vi "Update PhXP Parameters.vi"(8 "error in (no error)":errorcluster, 11 "VI in":refnum<vi>) -> (0 "error out":errorcluster, 2 "tau*":dbl[unit], 3 "f0":dbl[unit])   [LabVIEW 2019]
uses:
  Phasor Explorer Phasor Parameters.ctl
  Phasor Calculation Type.ctl
  Phasor Type.ctl
  Phasor Explorer Gate Parameters.ctl
  Gate Type.ctl
  SEPXP Gate Parameter to Adjust.ctl
  Phasor Explorer Decay Parameters.ctl
  IRF Model.ctl
  Phasor Explorer Display Parameters.ctl
  Type of Series.ctl
panel:
  in  "Edit User-defined Gate":bool
  in  "Phasor Explorer Display Parameters":T1={"# Points"=1, "Ramp Type"=enum."Linear", "Type of Series"=enum."1-Exp Decays", "Min tau"=0.0, "Max tau"=0.0, "Include 0"=FALSE, "Include Infinity"=FALSE} {"Min tau" min=0.0; "Max tau" min=0.0; "# Points" min=1 step=1}
  in  "Phasor Explorer Decay & IRF Parameters":T3 {"Lifetime" min=0.0; "Laser Period" min=0.0}
  in  "Gate Parameter to Adjust":T5 caption="Parameter to adjust"
  in  "Phasor Explorer Gate Parameters":T6={"First Gate Start"=0.0, "Use Gate Center"=FALSE, "Gate Width"=0.0, "Gate Step"=0.0, "# Gates"=1.0, "Gate Type"=enum."Square", "Edge Width"=0.0, "Top Slope"=0.0, "Reversed Sawtooth?"=FALSE, "Analytical Computation"=FALSE, "Tolerance"=1.0, "Integration"=enum."Item 0", "# Steps"=1.0, "Type of User-defined Function"=enum."Gate"} {"# Steps" min=0.0; "Tolerance" min=0.0; "Top Slope" min=0.0; "Edge Width" min=0.0; "Gate Step" min=0.0; "# Gates" min=1.0 step=1.0; "Gate Width" min=0.0}
  in  "Phasor Explorer Phasor Parameters":T8={"Harmonic frequency"=0.0, "Use f* = 1/D Frequency"=FALSE, "Calibrated Phasor"=FALSE, "Calibration Lifetime"=1e-09, "Phasor Calculation"=enum."Direct Sum", "SEPL Type"=enum."UC", "# Gates"=1.0, "Square Gate Width"=1e-09, "Show Ticks"=FALSE} {"Square Gate Width" min=0.0; "# Gates" min=0.0; "Calibration Lifetime" min=0.0; "Harmonic frequency" min=0.0}
  in  "Match Laser Period":bool
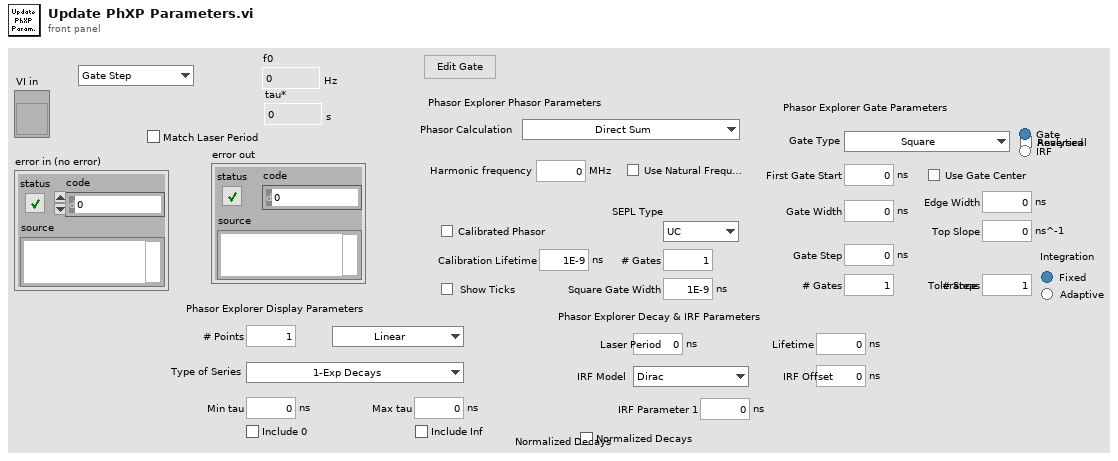
[diagram p1: front panel]
types:
  T1 = typedef "Phasor Explorer Display Parameters.ctl" = cluster{"# Points":i32, "Ramp Type":enum16{"Linear", "Logarithmic"}, "Type of Series":T2, "Min tau":dbl[unit], "Max tau":dbl[unit], "Include 0":bool, "Include Infinity":bool}
  T2 = typedef "Type of Series.ctl" = enum16{"1-Exp Decays", "Linear Combination of 1-Exp"}
  T3 = typedef "Phasor Explorer Decay Parameters.ctl" = cluster{"Lifetime":dbl[unit], "IRF Offset":dbl[unit], "Laser Period":dbl[unit], "Normalized Decays":bool, "IRF Model":T4, "IRF Parameter 1":dbl[unit]}
  T4 = typedef "IRF Model.ctl" = enum16{"Dirac", "Exponential"}
  T5 = typedef "SEPXP Gate Parameter to Adjust.ctl" = enum16{"Gate Step", "# Gates"}
  T6 = typedef "Phasor Explorer Gate Parameters.ctl" = cluster{"First Gate Start":dbl[unit], "Use Gate Center":bool, "Gate Width":dbl[unit], "Gate Step":dbl[unit], "# Gates":dbl, "Gate Type":T7, "Edge Width":dbl[unit], "Top Slope":dbl[unit], "Reversed Sawtooth?":bool, "Analytical Computation":bool, "Tolerance":dbl, "Integration":enum32{"Item 0", "Item 1"}, "# Steps":dbl, "Type of User-defined Function":enum32{"Gate", "IRF"}}
  T7 = typedef "Gate Type.ctl" = enum16{"Square", "Finite Edge Square", "Finite Edge, Tilted Top Square", "Triangle", "Sawtooth", "User-defined"}
  T8 = typedef "Phasor Explorer Phasor Parameters.ctl" = cluster{"Harmonic frequency":dbl[unit], "Use f* = 1/D Frequency":bool, "Calibrated Phasor":bool, "Calibration Lifetime":dbl[unit], "Phasor Calculation":T9, "SEPL Type":T10, "# Gates":dbl, "Square Gate Width":dbl[unit], "Show Ticks":bool}
  T9 = typedef "Phasor Calculation Type.ctl" = enum16{"Direct Sum", "Analytical Formula"}
  T10 = typedef "Phasor Type.ctl" = enum16{"UC", "L_N", "L_N[W]"}
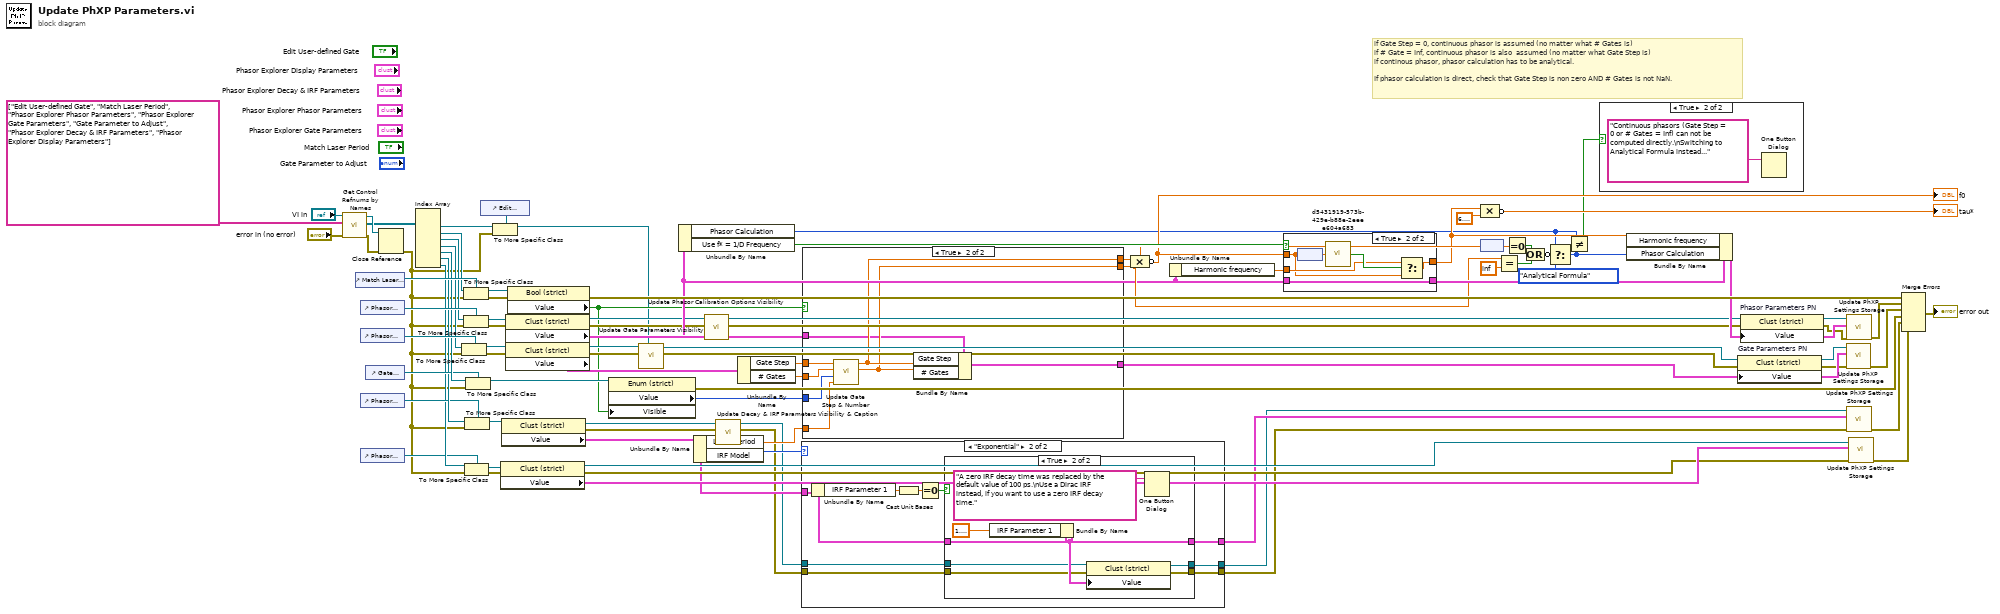
[diagram p0: block diagram]
diagram:
  # "if Gate Step = 0, continuous phasor is assumed (no matter what # Gates is)\nif # Gate = Inf, continuous phasor is also  assumed (no matter what Gate Step is)\nif continous phasor, phasor calculation has to be analytical.\n\nIf phasor calculation is direct, check that Gate Step is non zero AND # Gates is not NaN."
  n1 = call "Get Control Refnums by Names.vi"("error in"="error in (no error)", "Control Labels"=string[] ["Edit User-defined Gate", "Match Laser Period", "Phasor Explorer Phasor Parameters", "Phasor Explorer Gate Parameters", "Gate Parameter to Adjust", "Phasor Explorer Decay & IRF Parameters", "Phasor Explorer Display Parameters"], "VI  Ref"="VI in") -> ("error out"=w5:errorcluster, "Ctl Refnums"=w86:refnum<vi>[], "VI  Ref (out)"=w87:refnum<vi>)  [unwired: 5 in, 1 out]
  n2 = control-ref of="Match Laser Period"() -> (w79:refnum<vi>)
  n3 = control-ref of="Phasor Explorer Phasor Parameters"() -> (w82:refnum<vi>)
  n4 = control-ref of="Phasor Explorer Gate Parameters"() -> (w81:refnum<vi>)
  n5 = control-ref of="Phasor Explorer Decay & IRF Parameters"() -> (w54:refnum<vi>)
  n6 = control-ref of="Phasor Explorer Display Parameters"() -> (w33:refnum<vi>)
  n7 = control-ref of="Gate Parameter to Adjust"() -> (w73:refnum<vi>)
  n8 = Close Reference(reference=w87, error in (no error)=w5) -> (error out=w2:errorcluster)
  n9 = Index Array(array=w86) -> (element #1=w4:refnum<vi>, element #2=w58:refnum<vi>, element #3=w57:refnum<vi>, element #4=w56:refnum<vi>, element #5=w75:refnum<vi>, element #6=w55:refnum<vi>, element #7=w34:refnum<vi>)  [unwired: 7 in]
  n10 = To More Specific Class(target class=w81, reference=w56, error in=w2) -> (specific class reference=w62:refnum<vi>, error out=w61:errorcluster)
  n11 = To More Specific Class(target class=w79, reference=w58, error in=w2) -> (specific class reference=w78:refnum<vi>, error out=w77:errorcluster)
  n12 = To More Specific Class(target class=w82, reference=w57, error in=w2) -> (specific class reference=w64:refnum<vi>, error out=w63:errorcluster)
  n13 = To More Specific Class(target class=w33, reference=w34, error in=w2) -> (specific class reference=w32:refnum<vi>, error out=w31:errorcluster)
  n14 = To More Specific Class(target class=w54, reference=w55, error in=w2) -> (specific class reference=w53:refnum<vi>)  [unwired: 1 out]
  n15 = To More Specific Class(target class=w73, reference=w75, error in=w2) -> (specific class reference=w74:refnum<vi>)  [unwired: 1 out]
  n16 = control-ref of="Edit User-defined Gate"() -> (w3:refnum<vi>)
  n17 = To More Specific Class(target class=w3, reference=w4, error in=w2) -> (specific class reference=w1:refnum<vi>)  [unwired: 1 out]
  n18 = property class="Clust (strict)"(reference=w32, error in=w31) -> (reference out=w28:refnum<vi>, error out=w26:errorcluster, "Value"=w27:T1)
  n19 = property class="Clust (strict)"(reference=w53) -> (reference out=w22:refnum<vi>, error out=w8:errorcluster, "Value"=w24:T3)  [unwired: 1 in]
  n20 = property class="Clust (strict)"(reference=w64, error in=w63) -> (reference out=w16:refnum<vi>, error out=w14:errorcluster, "Value"=w42:T8)
  n21 = property class="Clust (strict)"(reference=w62, error in=w61) -> (reference out=w35:refnum<vi>, error out=w12:errorcluster, "Value"=w51:T6)
  n22 = property class="Bool (strict)"(reference=w78, error in=w77) -> (error out=w76:errorcluster, "Value"=w6:bool)  [unwired: 1 out]
  n23 = property class="Enum (strict)"(reference=w74, "Visible"=w6) -> (error out=w71:errorcluster, "Value"=w72:T5)  [unwired: 1 in, 1 out]
  n24 = call "Update Gate Parameters Visibility.vi"("Edit User-defined Gate"=w1, "error in (no error)"=w12, "Phasor Explorer Gate Parameters in"=w35) -> ("error out"=w11:errorcluster, "Phasor Explorer Gate Parameters out"=w10:refnum<vi>)  [unwired: 7 in]
  n25 = Unbundle By Name(w42) -> ("Phasor Calculation"=w19:T9, "Use f* = 1/D Frequency"=w85:bool)
  n26 = Unbundle By Name(w24) -> ("Laser Period"=w52:dbl[unit], "IRF Model"=w25:T4)
  n27 = call "Update Phasor Calibration Options Visibility.vi"("Error In"=w14, "Phasor Explorer Phasor Parameters Refnum in"=w16) -> ("Error Out"=w13:errorcluster, "Phasor Explorer Phasor Parameters Refnum out"=w15:refnum<vi>)  [unwired: 8 in]
  n28 = call "Update Decay & IRF Parameters Visibility & Caption.vi"("error in (no error)"=w8, "Phasor Explorer Decay & IRF Parameters in"=w22) -> ("error out"=w7:errorcluster, "Phasor Explorer Decay & IRF Parameters out"=w9:refnum<vi>)  [unwired: 8 in]
  n29 = Unbundle By Name(w51) -> ("Gate Step"=w60:dbl[unit], "# Gates"=w59:dbl)
  n30 = case shown="\"Exponential\"" w25 {
    tunnel: w24 -> [w93 w99]
    tunnel: [w93 w98] -> w23
    tunnel: w9 -> [w92 w97]
    tunnel: [w92 w96] -> w21
    tunnel: w7 -> [w91 w95]
    tunnel: [w91 w94] -> w20
    frame "Dirac", Default {
    }
    frame "Exponential" {
      n31 = Unbundle By Name(w99) -> ("IRF Parameter 1"=w102:dbl[unit])
      n32 = Cast Unit Bases(0:w102) -> (2:w101:dbl)  [unwired: 1 in]
      n33 = Equal To 0?(x=w101) -> (x = 0?=w100:bool)
      n34 = case shown="True" w100 {
        tunnel: w99 -> [w105 w112]
        tunnel: [w105 w110] -> w98
        tunnel: w97 -> [w104 w109]
        tunnel: [w104 w108] -> w96
        tunnel: w95 -> [w103 w107]
        tunnel: [w103 w106] -> w94
        frame False {
        }
        frame True {
          n35 = Bundle By Name(cluster=w112, "IRF Parameter 1"=dbl[unit] 1.0000000000000002e-10) -> (w110:T3)
          n36 = property class="Clust (strict)"(reference=w109, error in=w107, "Value"=w110) -> (reference out=w108:refnum<vi>, error out=w106:errorcluster)
          n37 = One Button Dialog(message="A zero IRF decay time was replaced by the default value of 100 ps.\nUse a Dirac IRF instead, if you want to use a zero IRF decay time.") -> ()  [unwired: 1 in, 1 out]
        }
      }
    }
  }
  n38 = case shown="True" w6 {
    tunnel: w52 -> [_ w118]
    tunnel: [w116 w124] -> w49
    tunnel: [w115 w123] -> w48
    tunnel: w72 -> [_ w122]
    tunnel: w60 -> [w116 w121]
    tunnel: w59 -> [w115 w120]
    tunnel: w51 -> [w114 w119]
    tunnel: [w114 w117] -> w37
    frame False {
    }
    frame True {
      n39 = call "Update Gate Step & Number.vi"("Period"=w118, "Value to Update"=w122, "# Gates in"=w120, "Gate Step in"=w121) -> ("# Gates out"=w123:dbl, "Gate Step out"=w124:dbl[unit])  [unwired: 6 in]
      n40 = Bundle By Name(cluster=w119, "Gate Step"=w124, "# Gates"=w123) -> (w117:T6)
    }
  }
  n41 = Compound Arithmetic op=MULTIPLY(w49, w48) -> (invert w43:dbl[unit])
  "f0" <- w43
  n42 = Unbundle By Name(w42) -> ("Harmonic frequency"=w41:dbl[unit])
  n43 = case shown="True" w85 {
    tunnel: w43 -> [_ w129]
    tunnel: [w125 w128] -> w47
    tunnel: w42 -> [w126 w132]
    tunnel: [w126 w132] -> w50
    tunnel: w41 -> [w125 w130]
    frame False {
    }
    frame True {
      # "update harmonic frequency"
      n44 = node(w129) -> (w127:dbl)
      n45 = call "d5431919-573b-429e-b88e-2eeee604a683.vi"("Number"=w127) -> ("Is NaN or Inf?"=w131:bool)  [unwired: 8 in]
      n46 = Select(t=w130, s=w131, f=w129) -> (s? t:f=w128:dbl[unit])
    }
  }
  n47 = node(w49) -> (w70:dbl)
  n48 = Compound Arithmetic op=MULTIPLY(w47, 6.283185307179586) -> (invert →"tau*":dbl[unit])
  n49 = Equal?(x=w48, y=inf) -> (x = y?=w67:bool)
  n50 = Equal To 0?(x=w70) -> (x = 0?=w68:bool)
  n51 = Compound Arithmetic op=OR(w68, w67) -> (invert w66:bool)
  n52 = Select(t=w19, s=w66, f=Phasor_Calculation_Type."Analytical Formula") -> (s? t:f=w18:T9)
  n53 = Not Equal?(x=w19, y=w18) -> (x != y?=w17:bool)
  n54 = case shown="True" w17 {
    frame False {
    }
    frame True {
      n55 = One Button Dialog(message="Continuous phasors (Gate Step = 0 or # Gates = Inf) can not be computed directly.\nSwitching to Analytical Formula instead...") -> ()  [unwired: 1 in, 1 out]
    }
  }
  n56 = Bundle By Name(cluster=w50, "Harmonic frequency"=w47, "Phasor Calculation"=w18) -> (w44:T8)
  n57 = property on="Gate Parameters PN" class="Clust (strict)"(reference=w10, error in=w11, "Value"=w37) -> (reference out=w38:refnum<vi>, error out=w36:errorcluster)
  n58 = property on="Phasor Parameters PN" class="Clust (strict)"(reference=w15, error in=w13, "Value"=w44) -> (reference out=w45:refnum<vi>, error out=w39:errorcluster)
  n59 = call "Update PhXP Settings Storage.vi"("Error In"=w36, "NewVal"=w37, "CtlRef"=w38) -> ("Error Out"=w40:errorcluster)  [unwired: 8 in]
  n60 = call "Update PhXP Settings Storage.vi"("Error In"=w39, "NewVal"=w44, "CtlRef"=w45) -> ("Error Out"=w46:errorcluster)  [unwired: 8 in]
  n61 = call "Update PhXP Settings Storage.vi"("Error In"=w20, "NewVal"=w23, "CtlRef"=w21) -> ("Error Out"=w30:errorcluster)  [unwired: 8 in]
  n62 = call "Update PhXP Settings Storage.vi"("Error In"=w26, "NewVal"=w27, "CtlRef"=w28) -> ("Error Out"=w29:errorcluster)  [unwired: 8 in]
  n63 = Merge Errors(w76, w46, w40, w71, w30, w29) -> (→"error out":errorcluster)
